vi "Start.vi"(8 "error in (no error)":errorcluster, 10 "Message in":refnum<class "StartMessage.lvclass">, 11 "ImageStack in":refnum<class "ImageStack.lvclass">) -> (0 "error out":errorcluster, 3 "ImageStack out":refnum<class "ImageStack.lvclass">)   [LabVIEW 2012, in "ImageStack.lvclass"]
doc: "This member function is called when the statemachine in the run.vi receives an 'start' command. It relays the message to all observers of the component.\n\nOverride this member function in your derived class if you need additional start functionality (but don't forget to call the parent method)."
uses:
  ImageStack.lvclass
  <vilib>/Distrio/Murmex/StartMessage/StartMessage.lvclass
  <vilib>/Distrio/Murmex/StartMessage/run mode enum.ctl
  ImageStack.lvclass/ImageStack.ctl
  <vilib>/Distrio/Murmex/Murmex/Murmex.lvclass
panel:
  # "This member function is called when the statemachine in the run.vi receives an 'start' command. It relays the message to all observers of the component.\n\nOverride this member function in your derived class if you need additional start functionality (but don't forget to call the parent method)."
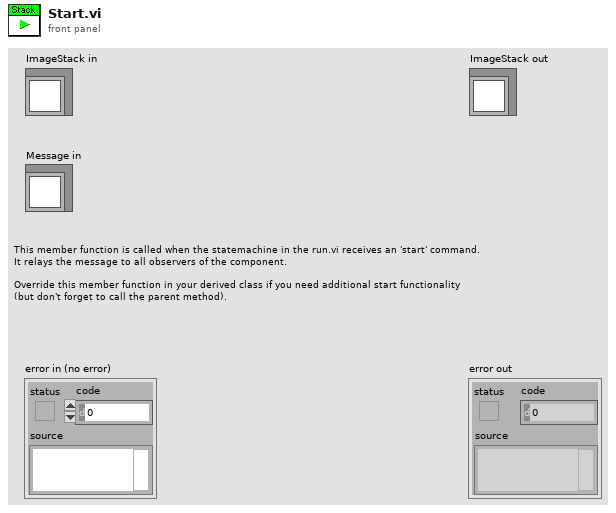
[diagram p1: front panel]
types:
  T1 = typedef "Murmex.lvlib/StartMessage.lvclass/run mode enum.ctl" = enum16{"infinite", "finite"}
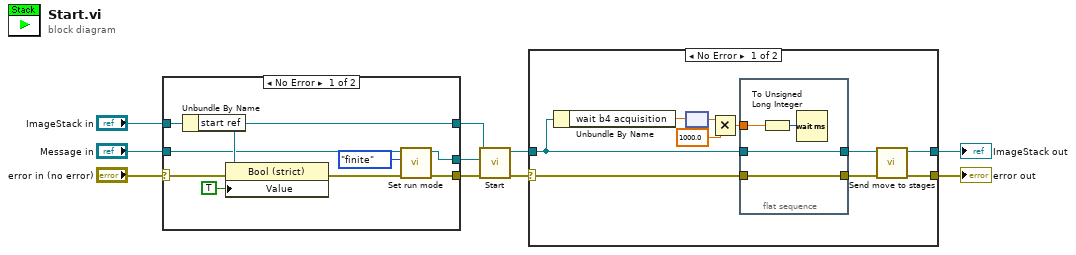
[diagram p0: block diagram]
diagram:
  n1 = case shown="No Error" "error in (no error)" {
    selector: "error in (no error)" -> [w18 w20]
    tunnel: "ImageStack in" -> [w11 w22]
    tunnel: "Message in" -> [w15 w21]
    tunnel: [w13 w21] -> w7
    tunnel: [w12 w20] -> w6
    tunnel: [w11 w22] -> w5
    frame No Error {
      n2 = Unbundle By Name(w11) -> ("start ref"=w19:refnum<vi>)
      n3 = property class="Bool (strict)"(reference=w19, error in=w18, "Value"=TRUE) -> (error out=w16:errorcluster)  [unwired: 1 out]
      n4 = call <vilib>:"Set run mode.vi"("error in (no error)"=w16, "run mode"=run_mode_enum."finite", "StartMessage in"=w15) -> ("error out"=w12:errorcluster, "StartMessage out"=w13:refnum<class "StartMessage.lvclass">)  [unwired: 7 in]
    }
    frame Error {
    }
  }
  n5 = call-parent "Start.vi"("error in (no error)"=w6, "Message in"=w7, "Murmex in"=w5) -> ("error out"=w4:errorcluster, "Murmex out"=w3:refnum<class "ImageStack.lvclass">)  [unwired: 7 in]
  n6 = case shown="No Error" w4 {
    selector: w4 -> [w28 w37]
    tunnel: w3 -> [w27 w38]
    tunnel: [w24 w37] -> w2
    tunnel: [w23 w38] -> w1
    frame No Error {
      n7 = Unbundle By Name(w27) -> ("wait b4 acquisition"=w32:dbl[unit])
      n8 = node(w32) -> (w31:dbl)
      n9 = Multiply(x=w31, y=1000.0) -> (x*y=w29:dbl)
      n10 = flat-sequence {
        tunnel: w29 -> [w35]
        tunnel: w28 -> [w34]
        tunnel: w27 -> [w33]
        tunnel: [w34] -> w25
        tunnel: [w33] -> w26
        frame #0 {
          n11 = To Unsigned Long Integer(number=w35) -> (unsigned 32bit integer=w36:u32)
          n12 = Wait (ms)(milliseconds to wait=w36) -> ()  [unwired: 1 out]
        }
      }
      n13 = call-dynamic "Send move to stages.vi"("error in (no error)"=w25, "ImageStack in"=w26) -> ("error out"=w24:errorcluster, "ImageStack out"=w23:refnum<class "ImageStack.lvclass">)  [unwired: 8 in]
    }
    frame Error {
    }
  }
  "error out" <- w2
  "ImageStack out" <- w1
